vi "Set Response Configuration.vi"(7 "Connection Name":string, 8 "error in (no error)":errorcluster, 10 "Response Configuration":T1, 11 "Module ID":i32=-1) -> (0 "error out":errorcluster)   [LabVIEW 2017, in "SSH.lvlib"]
doc: "<b>Note</b>: This VI was renamed by the DQMH Rename Event utility. Make sure the VI Description is updated to reflect the new event name, then delete this comment.\n\nSets the string to return a stream on\n_____\nCreated using Delacor QMH Event Scripter 4.2.1.88."
uses:
  SSH.lvlib
  Response Configuration.ctl
  Set Response Configuration Argument--cluster.ctl
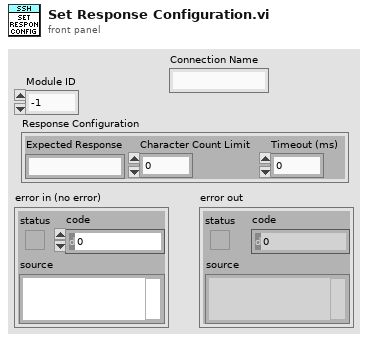
[diagram p1: front panel]
types:
  T1 = typedef "SSH.lvlib/Response Configuration.ctl" = cluster{"Expected Response":string, "Character Count Limit":i32, "Timeout (ms)":u32}
  T2 = typedef "SSH.lvlib/Set Response Configuration Argument--cluster.ctl" = cluster{"Module ID":i32, "Response Configuration":T1}
  T3 = typedef "SSH.lvlib/Request Events--cluster.ctl" = cluster{"Stop Module":refnum<user-event>, "Show Panel":refnum<user-event>, "Hide Panel":refnum<user-event>, "Show Diagram":refnum<user-event>, "Get Module Execution Status":refnum<user-event>, "Write Command":refnum<user-event>, "Set Response Configuration":refnum<user-event>}
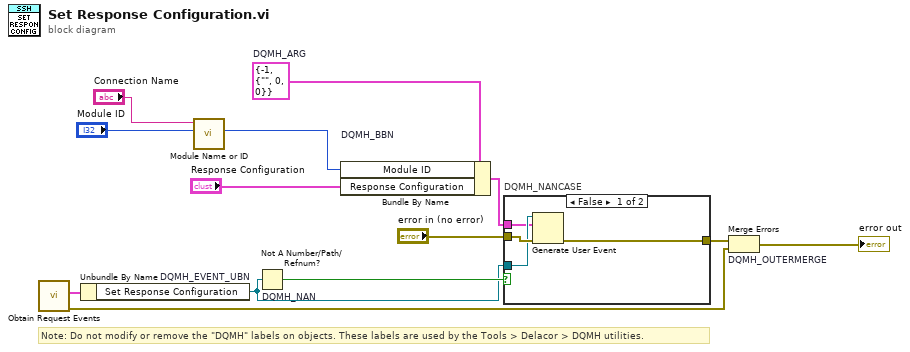
[diagram p0: block diagram]
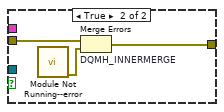
[diagram p2: hidden frame]
diagram:
  w7 = T2 {"Module ID"=-1, "Response Configuration"={"Expected Response"="", "Character Count Limit"=0, "Timeout (ms)"=0}}  # DQMH_ARG
  # "Note: Do not modify or remove the \"DQMH\" labels on objects. These labels are used by the Tools > Delacor > DQMH utilities."
  n1 = call "Obtain Request Events.vi"() -> ("error out"=w5:errorcluster, "SSH Request Events"=w4:T3)  [unwired: 10 in]
  n2 = Unbundle By Name "DQMH_EVENT_UBN"(w4) -> ("Set Response Configuration"=w9:refnum<user-event>)
  n3 = call "Module Name or ID.vi"("Module ID in"="Module ID", "Connection Name"="Connection Name") -> ("Module ID out"=w2:i32)  [unwired: 9 in]
  n4 = Not A Number/Path/Refnum? "DQMH_NAN"(number/path/refnum=w9) -> (NaN/Path/Refnum?=w10:bool)
  n5 = Bundle By Name "DQMH_BBN"(cluster=w7, "Module ID"=w2, "Response Configuration"="Response Configuration") -> (w11:T2)
  n6 = case "DQMH_NANCASE" shown="False" w10 {
    tunnel: "error in (no error)" -> [w17 w20]
    tunnel: [w16 w19] -> w8
    tunnel: w9 -> [w15 _]
    tunnel: w11 -> [w14 _]
    frame False {
      n7 = Generate User Event(user event=w15, event data cluster=w14, error in=w17) -> (error out=w16:errorcluster)  [unwired: 1 in, 1 out]
    }
    frame True {
      n8 = call "Module Not Running--error.vi"() -> ("error out"=w18:errorcluster)  [unwired: 11 in]
      n9 = Merge Errors "DQMH_INNERMERGE"(w20, w18) -> (w19:errorcluster)
    }
  }
  n10 = Merge Errors "DQMH_OUTERMERGE"(w8, w5) -> (→"error out":errorcluster)
